vi "FlatToRichcif_waveformmonitor_Waveforms.vi"(5 "OutputClusterType":T1, 11 "InputCluster":T3) -> (3 "OutputCluster":T1)   [LabVIEW 2021, in "CIFWaveformMonitor_server.lvlib"]
uses:
  CIFWaveformMonitor_server.lvlib
  cif_waveformmonitor_Waveforms_Flat.ctl
  cif_waveformmonitor_Waveform_Flat.ctl
  cif_waveformmonitor_Waveforms.ctl
  cif_waveformmonitor_Waveform.ctl
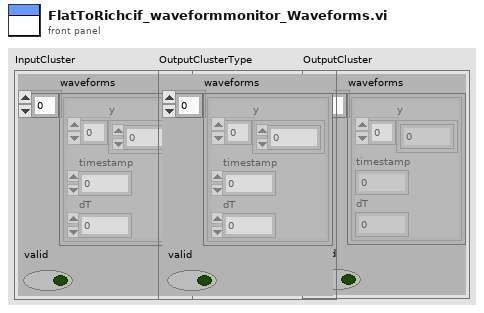
[diagram p1: front panel]
types:
  T1 = typedef "CIFWaveformMonitor_server.lvlib/cif_waveformmonitor_Waveforms.ctl" = cluster{"waveforms":T2[], "valid":bool}
  T2 = typedef "CIFWaveformMonitor_server.lvlib/cif_waveformmonitor_Waveform.ctl" = cluster{"y":dbl[], "timestamp":u64, "dT":dbl}
  T3 = typedef "CIFWaveformMonitor_server.lvlib/cif_waveformmonitor_Waveforms_Flat.ctl" = cluster{"waveforms":T4[], "valid":bool}
  T4 = typedef "CIFWaveformMonitor_server.lvlib/cif_waveformmonitor_Waveform_Flat.ctl" = cluster{"y":dbl[], "timestamp":u64, "dT":dbl}
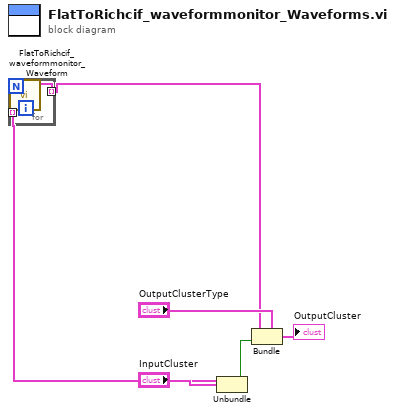
[diagram p0: block diagram]
diagram:
  n1 = Unbundle "Unbundle"("InputCluster") -> ("waveforms"=w3:T4[], "valid"=w1:bool)
  n2 = for {
    tunnel: w3 -> [w8] mode=indexing
    tunnel: [w7] -> w2 mode=indexing
    n3 = call "FlatToRichcif_waveformmonitor_Waveform.vi"("InputCluster"=w8) -> ("OutputCluster"=w7:T2)  [unwired: 10 in]
  }
  n4 = Bundle "Bundle"(cluster="OutputClusterType", "waveforms"=w2, "valid"=w1) -> (→"OutputCluster":T1)
